vi "SVPO TDMS Write SGL Array (N Ch N Info).vi"(0 "tdms file":refnum<k34>, 1 "write channel properties? (T)":bool=TRUE, 5 "group name in":string="Waveform", 7 "channel names in":string[](array[string]), 9 "scaled signals [EU]":sgl[][](array[numeric]), 11 "sampling rate [Hz]":dbl=1.0, 12 "unit labels":string[](array[string])) -> (4 "tdms file out":refnum<k34>, 6 "group name out":string, 8 "channel names out":string[](array[string]))   [LabVIEW 2017]
doc: "Writes single-precision waveform or scaled array data to the specified .tdms file in a format specific to the polymorphic instance. Use this VI on embedded targets that have limited computational resources. Wire data to the <B>scaled signal [EU]</B> input to determine the polymorphic instance to use or manually select the instance."
uses:
  <vilib>/addons/_NISVFA/_Shared subVIs/Controls/NI Channel Properties.ctl
  <vilib>/addons/_NISVFA/_Shared subVIs/Controls/LV Datatypes.ctl
  <vilib>/addons/_NISVFA/_Shared subVIs/Controls/svc_X-Axis Units.ctl
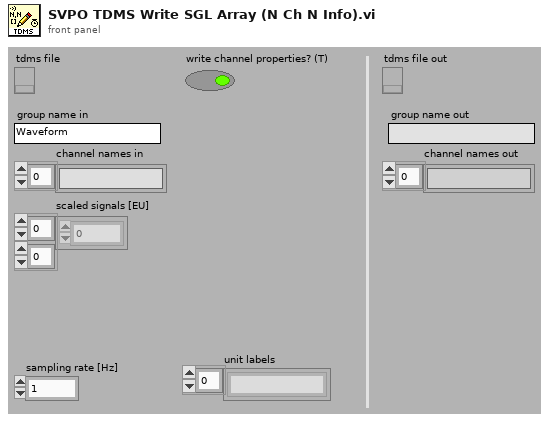
[diagram p1: front panel]
types:
  T1 = typedef "svc_X-Axis Units.ctl" = u16
  T2 = typedef "LV Datatypes.ctl" = i32
  T3 = typedef "NI Channel Properties.ctl" = u16
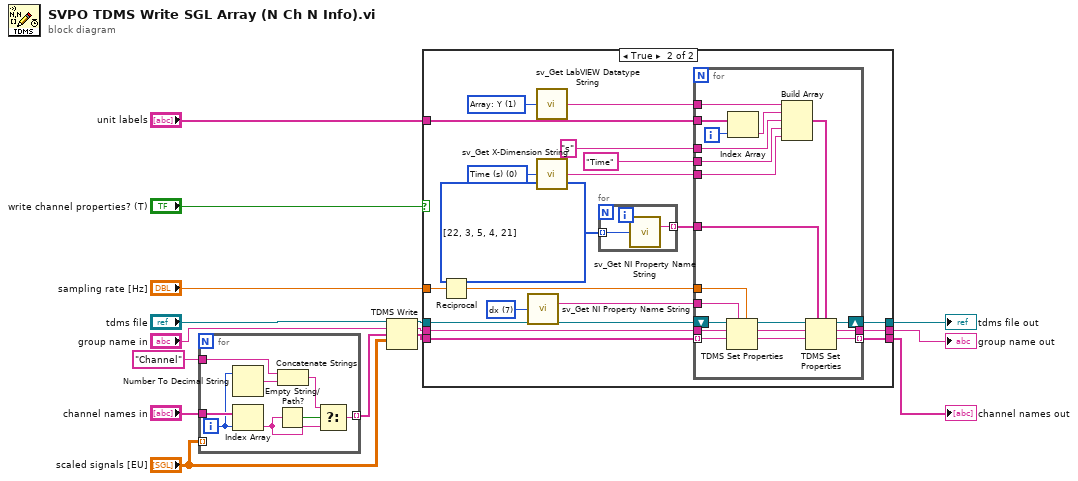
[diagram p0: block diagram]
diagram:
  n1 = for {
    tunnel: "channel names in" -> [w23]
    tunnel: [w22] -> w5 mode=indexing
    tunnel: "Channel" ("string") -> [w17]
    tunnel: "scaled signals [EU]" -> [_] mode=indexing
    i -> [w20]
    n2 = Number To Decimal String(number=w20) -> (decimal integer string=w19:string)  [unwired: 1 in]
    n3 = Index Array(array=w23, index=w20) -> (element=w16:string)
    n4 = Empty String/Path?(string/path=w16) -> (empty?=w21:bool)
    n5 = Concatenate Strings(w17, w19) -> (w18:string)
    n6 = Select(t=w18, s=w21, f=w16) -> (s? t:f=w22:string)
  }
  n7 = TDMS Write(0:"tdms file", 5:"group name in", 7:w5, 9:"scaled signals [EU]") -> (4:w14:refnum<k34>, 6:w12:string, 8:w11:string[])  [unwired: 2 in, 1 out]
  n8 = case shown="True" "write channel properties? (T)" {
    tunnel: [w26 w40] -> w9
    tunnel: w11 -> [w24 w44]
    tunnel: w12 -> [w25 w43]
    tunnel: w14 -> [w26 w42]
    tunnel: [w25 w45] -> w8
    tunnel: [w24 w41] -> w3
    tunnel: "sampling rate [Hz]" -> [_ w37]
    tunnel: "unit labels" -> [_ w30]
    frame False {
    }
    frame True {
      w33 = T1 0 items=["Time (s)"=0, "Frequency-CB (Hz)"=1, "Frequency-CPB (Hz)"=1248, "Frequency-Arbitrary (Hz)"=2357, "Quefrency (s)"=2, "Revolutions (rev)"=3, "Order"=4, "Speed (RPM)"=11, "Speed (rad/s)"=21, "Index"=65535] ("x-axis units")
      w32 = T2 1 items=["String"=-2, "Boolean"=-1, "Scalar: y"=0, "Array: Y"=1, "Waveform: t0, dt, Y, variant"=2, "Cluster: x0, dx, Y"=3, "Cluster: X, Y"=4, "Waterfall"=5, "Colormap"=6] ("LabVIEW datatype")
      w35 = T3[] [22, 3, 5, 4, 21] items=["Channel name", "Channel description", "Y-axis label", "Y-axis unit string", "X-axis label", "X-axis unit string", "x0", "dx", "Number of samples", "X channel", "Filter settled", "dB reference", "Window", "Window parameter", "Window size", "FFT size", "Peak units", "Spectrum type", "Magnitude scale", "Spectral density", "Sensor sensitivity (mV/EU)", "X-axis domain", "LabVIEW datatype"]
      w39 = T3 7 items=["Channel name", "Channel description", "Y-axis label", "Y-axis unit string", "X-axis label", "X-axis unit string", "x0", "dx", "Number of samples", "X channel", "Filter settled", "dB reference", "Window", "Window parameter", "Window size", "FFT size", "Peak units", "Spectrum type", "Magnitude scale", "Spectral density", "Sensor sensitivity (mV/EU)", "X-axis dimension", "LabVIEW datatype", "Function type", "Function subtype"] ("property")
      n9 = Reciprocal(x=w37) -> (1/x=w36:dbl)
      n10 = call <vilib>:"sv_Get NI Property Name String.vi"("property"=w39) -> ("TDMS property name"=w38:string)  [unwired: 13 in, 1 out]
      n11 = call <vilib>:"sv_Get LabVIEW Datatype String.vi"("LabVIEW datatype"=w32) -> ("datatype string"=w31:string)  [unwired: 4 in]
      n12 = call <vilib>:"sv_Get X-Dimension String.vi"("x-axis units"=w33) -> ("x-domain string"=w27:string)  [unwired: 4 in]
      n13 = for {
        tunnel: [w47] -> w34 mode=indexing
        tunnel: w35 -> [w46] mode=indexing
        n14 = call <vilib>:"sv_Get NI Property Name String.vi"("property"=w46) -> ("TDMS property name"=w47:string)  [unwired: 13 in, 1 out]
      }
      n15 = for {
        tunnel: [w56] -> w45
        tunnel: w44 -> [w59] mode=indexing
        tunnel: w43 -> [w60]
        shift-right: [w66] -> w40
        shift-left: w42 -> [w64]
        tunnel: [w65] -> w41 mode=indexing
        tunnel: w38 -> [w58]
        tunnel: w36 -> [w57]
        tunnel: w34 -> [w55]
        tunnel: w31 -> [w54]
        tunnel: w30 -> [w52]
        tunnel: "s" ("group name") -> [w51]
        tunnel: "Time" ("channel name") -> [w50]
        tunnel: w27 -> [w49]
        i -> [w67]
        n16 = TDMS Set Properties(5:w57, 7:w58, 9:w59, 10:w60, 11:w64) -> (1:w61:string, 2:w62:string, 3:w63:refnum<k34>)  [unwired: 1 in, 1 out]
        n17 = Index Array(array=w52, index=w67) -> (element=w53:string)
        n18 = Build Array(w54, w53, w51, w50, w49) -> (w48:string[])
        n19 = TDMS Set Properties(5:w48, 7:w55, 9:w61, 10:w62, 11:w63) -> (1:w65:string, 2:w56:string, 3:w66:refnum<k34>)  [unwired: 1 in, 1 out]
      }
    }
  }
  "tdms file out" <- w9
  "group name out" <- w8
  "channel names out" <- w3
